vi "Drive Motors.vi"(8 "Mode":enum16{"Init", "Run", "End"}(ring), 10 "Inputs":cluster{"Left Drive":dbl, "Right Drive":dbl}, 11 "PWM Module (DIO A)":T1={"PWM Module"=enum."Digital Module 2", "Unassigned"=enum."PWM 1", "Unassigned"=enum."PWM 2", "Right Motor"=enum."PWM 3", "Left Motor"=enum."PWM 4", "Unassigned"=enum."PWM 5", "Unassigned"=enum."PWM 6", "Unassigned"=enum."PWM 7", "Arm Motor"=enum."PWM 8", "Unassigned"=enum."PWM 9", "Unassigned"=enum."PWM 10", "Compressor"=enum."Relay 1", "Unassigned"=enum."Relay 2", "Unassigned"=enum."Relay 3", "Unassigned"=enum."Relay 4", "Unassigned"=enum."Relay 5", "Unassigned"=enum."Relay 6", "Unassigned"=enum."Relay 7", "Unassigned "=enum."Relay 8"}) -> ()   [LabVIEW 2013]
doc: "Use the VI to set the drive motors."
uses:
  Type Defs/PWM Module (DIO A).ctl
  <vilib>/Rock Robotics/SystemInterfaces/Typedef/FPGA_TypedefDigitalModule.ctl
  <vilib>/Rock Robotics/SystemInterfaces/DIO/FPGA_DIOPWMChannel.ctl
  <vilib>/Rock Robotics/SystemInterfaces/DIO/FPGA_DIORelayChannel.ctl
  <vilib>/Rock Robotics/WPI/SafetyOutput/WPI_SafetyOutputConfigMenu.ctl
  <vilib>/Rock Robotics/WPI/MotorControl/WPI_MotorControlOpen Victor.vi
  Team Code/Robot Global Data.vi
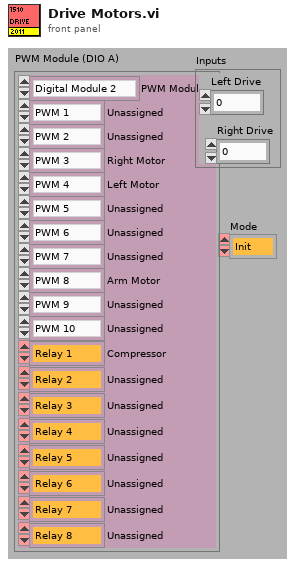
[diagram p1: front panel]
types:
  T1 = typedef "PWM Module (DIO A).ctl" = cluster{"PWM Module":T2, "Unassigned":T3, "Unassigned":T3, "Right Motor":T3, "Left Motor":T3, "Unassigned":T3, "Unassigned":T3, "Unassigned":T3, "Arm Motor":T3, "Unassigned":T3, "Unassigned":T3, "Compressor":T4, "Unassigned":T4, "Unassigned":T4, "Unassigned":T4, "Unassigned":T4, "Unassigned":T4, "Unassigned":T4, "Unassigned ":T4}
  T2 = typedef "FPGA_TypedefDigitalModule.ctl" = enum16{"Digital Module 1", "Digital Module 2"}
  T3 = typedef "FPGA_DIOPWMChannel.ctl" = enum8{"PWM 1", "PWM 2", "PWM 3", "PWM 4", "PWM 5", "PWM 6", "PWM 7", "PWM 8", "PWM 9", "PWM 10", "Invalid"}
  T4 = typedef "FPGA_DIORelayChannel.ctl" = enum8{"Relay 1", "Relay 2", "Relay 3", "Relay 4", "Relay 5", "Relay 6", "Relay 7", "Relay 8", "Invalid"}
  T5 = typedef "WPI_SafetyOutputConfigMenu.ctl" = enum16{"Enable", "Disable"}
  T6 = typedef "WPI_MotorControlDeviceRef.ctl" = cluster{"DeviceStatus":errorcluster, "Type":enum16{"PWM", "CAN"}, "PWM":cluster{"Digital Module":T2, "PWM Channel":T3, "DeadBand":T7}, "CAN":cluster{"Device Number":u8, "Control Mode":T8, "Semaphore":T9, "Max Vout":dbl}, "Invert":bool, "TransformRef":T10, "InvTransformRef":T10}
  T7 = typedef "WPI_PWMDeadband.ctl" = cluster{"Name":string, "maxPositivePwm":i32, "minPositivePwm":i32, "centerPwm":i32, "maxNegativePwm":i32, "minNegativePwm":i32, "angularRange":u16}
  T8 = typedef "WPI_CANJaguar_ControlMode.ctl" = enum8{"Percent VBus", "Current", "Speed", "Position", "Voltage"}
  T9 = typedef "Semaphore RefNum" = refnum<k1>
  T10 = typedef "WPI_PWMTransform_ConPane.ctl" = refnum<vi>
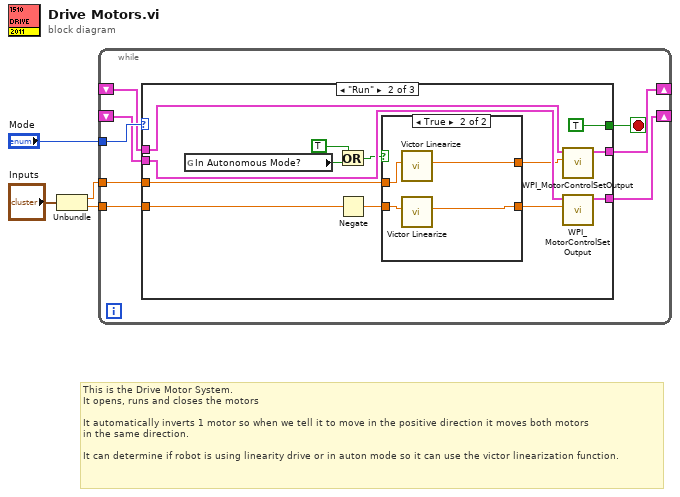
[diagram p0: block diagram]
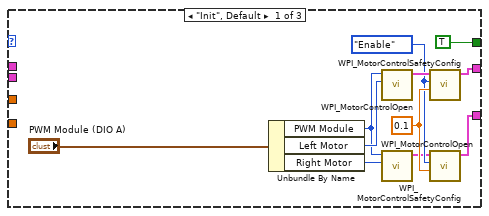
[diagram p2: hidden frame]
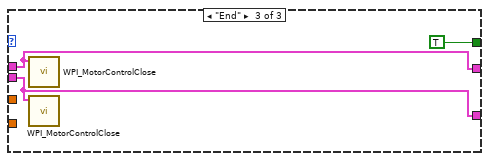
[diagram p4: hidden frame]
diagram:
  # "This is the Drive Motor System. \nIt opens, runs and closes the motors\n\nIt automatically inverts 1 motor so when we tell it to move in the positive direction it moves both motors\nin the same direction.\n\nIt can determine if robot is using linearity drive or in auton mode so it can use the victor linearization function."
  n1 = Unbundle("Inputs") -> ("Left Drive"=w3:dbl, "Right Drive"=w2:dbl)
  n2 = while {
    tunnel: "Mode" -> [w12]
    shift-right: [w11] -> _
    shift-left: _ -> [w10]
    shift-right: [w8] -> _
    shift-left: _ -> [w7]
    tunnel: w3 -> [w6]
    tunnel: w2 -> [w5]
    stop <- w9 stop-if-true
    n3 = case shown="\"Run\"" w12 {
      tunnel: [w19 w35 w44] -> w11
      tunnel: w10 -> [_ w34 w44]
      tunnel: [TRUE TRUE TRUE] -> w9
      tunnel: [w15 w32 w43] -> w8
      tunnel: w7 -> [_ w33 w43]
      tunnel: w6 -> [_ w30 _]
      tunnel: w5 -> [_ w31 _]
      frame "Init", Default {
        w18 = 0.1 ("timeout (s)")
        w17 = WPI_SafetyOutputConfigMenu."Enable" ("mode")
        n4 = Unbundle By Name("PWM Module (DIO A)") -> ("PWM Module"=w13:T2, "Left Motor"=w21:T3, "Right Motor"=w14:T3)
        n5 = call-poly <vilib>:"WPI_MotorControlOpen.vi"("PWM Channel"=w21, "Digital Module (Module 1)"=w13) -> ("MotorControlDeviceRef"=w20:T6)  [unwired: 5 in, 4 out]
        n6 = call-poly <vilib>:"WPI_MotorControlOpen.vi"("PWM Channel"=w14, "Digital Module (Module 1)"=w13) -> ("MotorControlDeviceRef"=w16:T6)  [unwired: 5 in, 4 out]
        n7 = call <vilib>:"WPI_MotorControlSafetyConfig.vi"("timeout (s)"=w18, "mode"=w17, "MotorControlDevRef"=w20) -> ("MotorControlDevRef"=w19:T6)  [unwired: 1 in, 7 out]
        n8 = call <vilib>:"WPI_MotorControlSafetyConfig.vi"("timeout (s)"=w18, "mode"=w17, "MotorControlDevRef"=w16) -> ("MotorControlDevRef"=w15:T6)  [unwired: 1 in, 7 out]
      }
      frame "Run" {
        n9 = global read "Robot Global Data.vi" "In Autonomous Mode?"() -> (w26:bool)
        n10 = Or(x=TRUE, y=w26) -> (x .or. y?=w25:bool)
        n11 = Negate(x=w31) -> (-x=w29:dbl)
        n12 = case shown="True" w25 {
          tunnel: [w38 w42] -> w27
          tunnel: [w37 w41] -> w28
          tunnel: w29 -> [w37 w40]
          tunnel: w30 -> [w38 w39]
          frame False {
          }
          frame True {
            n13 = call "Victor Linearize.vi"("Goal Speed"=w39) -> ("Output"=w42:dbl)  [unwired: 10 out]
            n14 = call "Victor Linearize.vi"("Goal Speed"=w40) -> ("Output"=w41:dbl)  [unwired: 10 out]
          }
        }
        n15 = call <vilib>:"WPI_MotorControlSetOutput.vi"("Output"=w27, "MotorControlDevRef"=w34) -> ("MotorControlDevRef"=w35:T6)  [unwired: 3 in, 6 out]
        n16 = call <vilib>:"WPI_MotorControlSetOutput.vi"("Output"=w28, "MotorControlDevRef"=w33) -> ("MotorControlDevRef"=w32:T6)  [unwired: 3 in, 6 out]
      }
      frame "End" {
        n17 = call <vilib>:"WPI_MotorControlClose.vi"("MotorControlDevRef"=w44) -> ()  [unwired: 1 in, 10 out]
        n18 = call <vilib>:"WPI_MotorControlClose.vi"("MotorControlDevRef"=w43) -> ()  [unwired: 1 in, 10 out]
      }
    }
  }
